vi "ep_Air Gap Torque.vi"(0 "phase voltage waveforms":waveform(dbl)[](array[waveform]), 1 "fundamental frequency [Hz]":dbl=50.0, 2 "reset? (F)":bool, 5 "current waveforms":waveform(dbl)[](array[waveform]), 7 "information":T2, 11 "error in (no error)":errorcluster, 12 "initial conditions":T1, 13 "stator resistance [ohms]":dbl) -> (4 "air-gap torque waveform [Nm]":waveform(dbl), 14 "final conditions":T1, 15 "error out":errorcluster)   [LabVIEW 2014, in "NI_EP_Motor Monitoring.lvlib"]
uses:
  <vilib>/addons/Electrical Power/Motor Monitoring/NI_EP_Motor Monitoring.lvlib
  <vilib>/addons/Electrical Power/Motor Monitoring/subVIs/ep_Initial Conditions for Air Gap.ctl
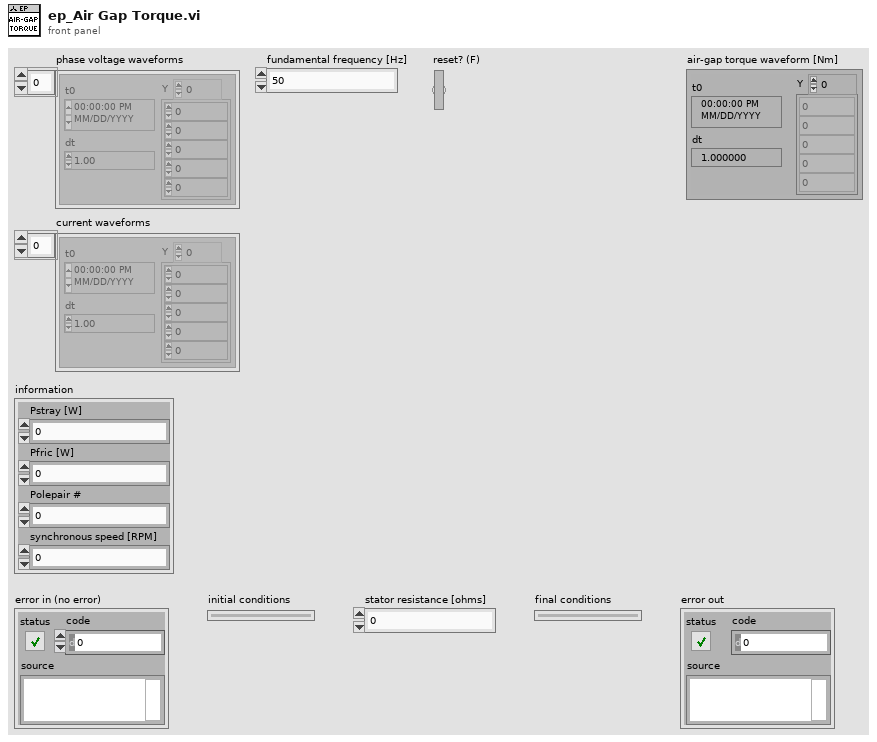
[diagram p1: front panel]
types:
  T1 = typedef "NI_EP_Motor Monitoring.lvlib/ep_Initial Conditions for Air Gap.ctl" = cluster{"integration state in A":cluster{"initial value":dbl, "initial integration":dbl}, "integration state in B":cluster{"initial value":dbl, "initial integration":dbl}, "integrated state A":dbl[], "integrated state B":dbl[], "previous length":i32, "loss and polepair":cluster{"Pstray [W]":dbl, "Pfric [W]":dbl, "Polepair #":i32, "synchronous speed [RPM]":dbl}, "expected timestamp":timestamp}
  T2 = cluster{"Pstray [W]":dbl, "Pfric [W]":dbl, "Polepair #":i32, "synchronous speed [RPM]":dbl}
  T3 = cluster{"initial value":dbl, "initial integration":dbl}
  T4 = cluster{"last value":dbl, "final integration":dbl}
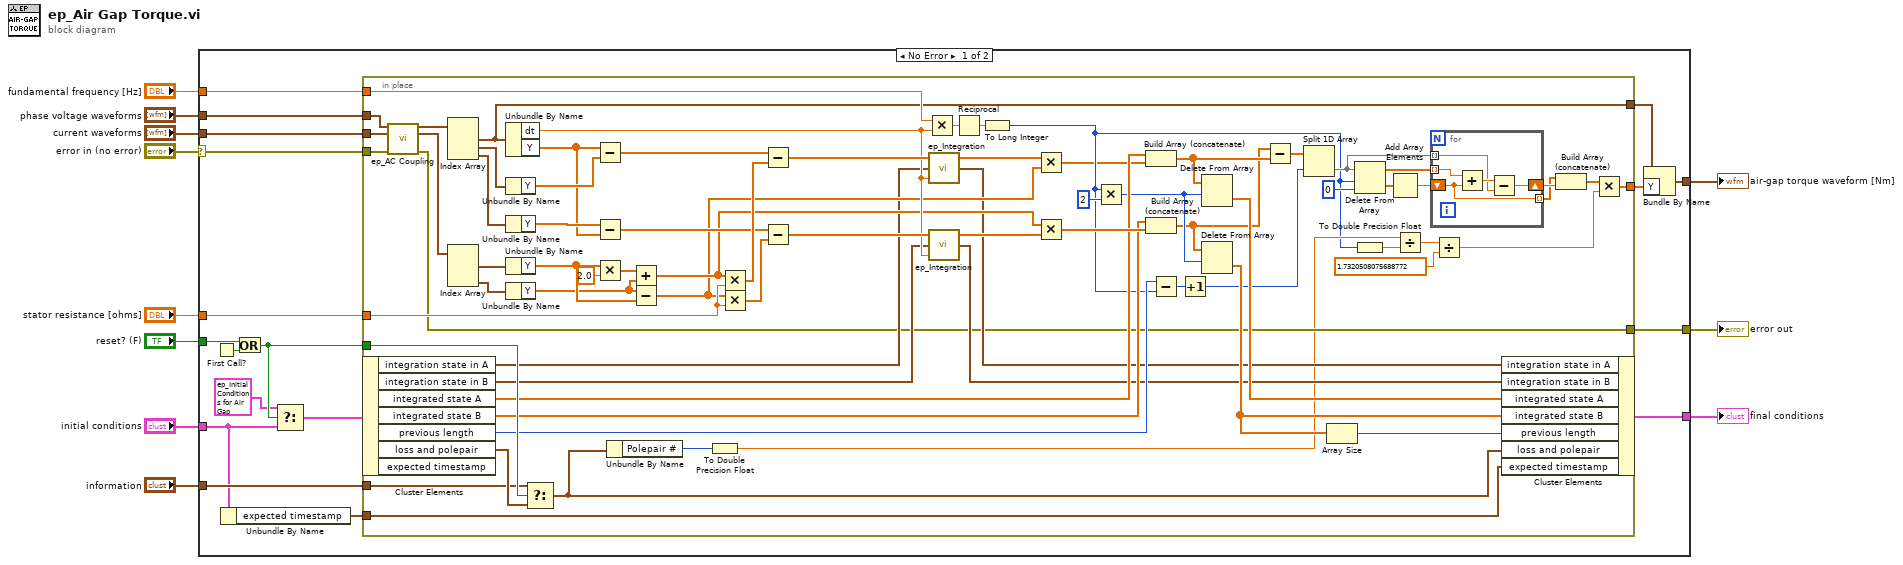
[diagram p0: block diagram]
diagram:
  n1 = case shown="No Error" "error in (no error)" {
    selector: "error in (no error)" -> [w27 w108]
    tunnel: [w19 w108] -> w10
    tunnel: "reset? (F)" -> [w28 _]
    tunnel: "current waveforms" -> [w26 _]
    tunnel: "phase voltage waveforms" -> [w25 _]
    tunnel: "stator resistance [ohms]" -> [w24 _]
    tunnel: "fundamental frequency [Hz]" -> [w23 _]
    tunnel: "initial conditions" -> [w14 _]
    tunnel: "information" -> [w20 _]
    tunnel: [w17 _] -> w3
    tunnel: [w16 _] -> w1
    frame No Error {
      n2 = First Call?() -> (First Call?: T/F=w29:bool)
      n3 = Unbundle By Name(w14) -> ("expected timestamp"=w13:timestamp)
      n4 = Or(x=w28, y=w29) -> (x .or. y?=w22:bool)
      n5 = Select(t=T1 {"integration state in A"={"initial value"=0.0, "initial integration"=0.0}, "integration state in B"={"initial value"=0.0, "initial integration"=0.0}, "integrated state A"=[], "integrated state B"=[], "previous length"=0, "loss and polepair"={"Pstray [W]"=0.0, "Pfric [W]"=0.0, "Polepair #"=0, "synchronous speed [RPM]"=0.0}, "expected timestamp"=timestamp(0 s since 1904-01-01)} ("initial conditions"), s=w22, f=w14) -> (s? t:f=w21:T1)
      n6 = in-place {
        in-place-border: w27 -> [w102]
        in-place-border: w26 -> [w101]
        in-place-border: w25 -> [w100]
        in-place-border: w24 -> [w85]
        in-place-border: w23 -> [w78]
        in-place-border: w22 -> [w74]
        in-place-border: w20 -> [w56]
        in-place-border: [w38] -> w18
        in-place-border: [w50] -> w19
        in-place-border: [w58] -> w15
        in-place-border: w13 -> [w51]
        n7 = in-place-cluster #1(w21) -> ("integration state in A"=w52:T3, "integration state in B"=w53:T3, "integrated state A"=w71:dbl[], "integrated state B"=w70:dbl[], "previous length"=w61:i32, "loss and polepair"=w60:T2)  [unwired: 1 out]
        n8 = call <vilib>:"ep_AC Coupling.vi"("phase voltage waveforms in"=w100, "current waveforms in"=w101, "error in (no error)"=w102) -> ("phase voltage waveforms out"=w99:waveform(dbl)[], "current waveforms out"=w98:waveform(dbl)[], "error out"=w50:errorcluster)  [unwired: 10 in]
        n9 = Index Array(array=w99) -> (element #1=w58:waveform(dbl), element #2=w97:waveform(dbl), element #3=w96:waveform(dbl))  [unwired: 3 in]
        n10 = Index Array(array=w98) -> (element #1=w94:waveform(dbl), element #3=w95:waveform(dbl))  [unwired: 3 in, 1 out]
        n11 = Unbundle By Name(w58) -> ("dt"=w79:dbl, "Y"=w91:dbl[])
        n12 = Unbundle By Name(w97) -> ("Y"=w93:dbl[])
        n13 = Unbundle By Name(w96) -> ("Y"=w92:dbl[])
        n14 = Unbundle By Name(w94) -> ("Y"=w88:dbl[])
        n15 = Unbundle By Name(w95) -> ("Y"=w87:dbl[])
        n16 = Select(t=w56, s=w74, f=w60) -> (s? t:f=w57:T2)
        n17 = Subtract(x=w91, y=w93) -> (x-y=w86:dbl[])
        n18 = Subtract(x=w92, y=w91) -> (x-y=w83:dbl[])
        n19 = Multiply(x=w88, y=2.0) -> (x*y=w90:dbl[])
        n20 = Unbundle By Name(w57) -> ("Polepair #"=w59:i32)
        n21 = Add(x=w90, y=w87) -> (x+y=w75:dbl[])
        n22 = Subtract(x=w87, y=w88) -> (x-y=w68:dbl[])
        n23 = To Double Precision Float(number=w59) -> (double precision float=w35:dbl)
        n24 = Multiply(x=w75, y=w85) -> (x*y=w84:dbl[])
        n25 = Multiply(x=w68, y=w85) -> (x*y=w82:dbl[])
        n26 = Subtract(x=w86, y=w84) -> (x-y=w81:dbl[])
        n27 = Subtract(x=w83, y=w82) -> (x-y=w80:dbl[])
        n28 = Multiply(x=w78, y=w79) -> (x*y=w77:dbl)
        n29 = call <vilib>:"ep_Integration.vi"("dt"=w79, "state in"=w52, "x(t)"=w81) -> ("state out"=w54:T4, "integrated x(t)"=w67:dbl[])  [unwired: 1 in]
        n30 = call <vilib>:"ep_Integration.vi"("dt"=w79, "state in"=w53, "x(t)"=w80) -> ("state out"=w55:T4, "integrated x(t)"=w66:dbl[])  [unwired: 1 in]
        n31 = Reciprocal(x=w77) -> (1/x=w76:dbl)
        n32 = To Long Integer(number=w76) -> (32bit integer=w33:i32)
        n33 = Multiply(x=w67, y=w68) -> (x*y=w32:dbl[])
        n34 = Multiply(x=w75, y=w66) -> (x*y=w73:dbl[])
        n35 = Multiply(x=w33, y=2) -> (x*y=w65:i32)
        n36 = Build Array (concatenate)(w71, w32) -> (w31:dbl[])
        n37 = Build Array (concatenate)(w70, w73) -> (w30:dbl[])
        n38 = Subtract(x=w61, y=w33) -> (x-y=w62:i32)
        n39 = Increment(x=w62) -> (x+1=w34:i32)
        n40 = Delete From Array(array=w31, length=w65) -> (deleted portion=w69:dbl[])  [unwired: 1 in, 1 out]
        n41 = Delete From Array(array=w30, length=w65) -> (deleted portion=w63:dbl[])  [unwired: 1 in, 1 out]
        n42 = Subtract(x=w30, y=w31) -> (x-y=w49:dbl[])
        n43 = Split 1D Array(array=w49, index=w34) -> (second subarray=w46:dbl[])  [unwired: 1 out]
        n44 = Array Size(array=w63) -> (size(s)=w64:i32)
        n45 = Delete From Array(array=w46, length=w33, index=0) -> (deleted portion=w47:dbl[], array with subset deleted=w45:dbl[])
        n46 = To Double Precision Float(number=w33) -> (double precision float=w41:dbl)
        n47 = Add Array Elements(numeric array=w47) -> (sum=w43:dbl)
        n48 = Divide(x=w35, y=w41) -> (x/y=w40:dbl)
        n49 = for {
          shift-right: [w104] -> w44
          shift-left: w43 -> [w103]
          tunnel: w46 -> [w105] mode=indexing
          tunnel: w45 -> [w107] mode=indexing
          tunnel: [w103] -> w42 mode=indexing
          n50 = Add(x=w107, y=w103) -> (x+y=w106:dbl)
          n51 = Subtract(x=w106, y=w105) -> (x-y=w104:dbl)
        }
        n52 = Divide(x=w40, y=1.7320508075688772) -> (x/y=w36:dbl)
        n53 = in-place-cluster #1("integration state in A"=w54, "integration state in B"=w55, "integrated state A"=w69, "integrated state B"=w63, "previous length"=w64, "loss and polepair"=w57, "expected timestamp"=w51) -> (w16:T1)
        n54 = Build Array (concatenate)(w42, w44) -> (w37:dbl[])
        n55 = Multiply(x=w37, y=w36) -> (x*y=w38:dbl[])
      }
      n56 = Bundle By Name(cluster=w15, "Y"=w18) -> (w17:waveform(dbl))
    }
    frame Error {
    }
  }
  "error out" <- w10
  "air-gap torque waveform [Nm]" <- w3
  "final conditions" <- w1
